vi "Project HMI.vi"() -> ()   [LabVIEW 2025]
panel:
  in  "Statistics":bool
  out "Statistics:":T1
  out "path":path
  out "temp file path":path
  in  "Save":bool
  out "?":T2 {"Temperature °C" scale=0.0..100.0}
  in  "ON/OFF":bool
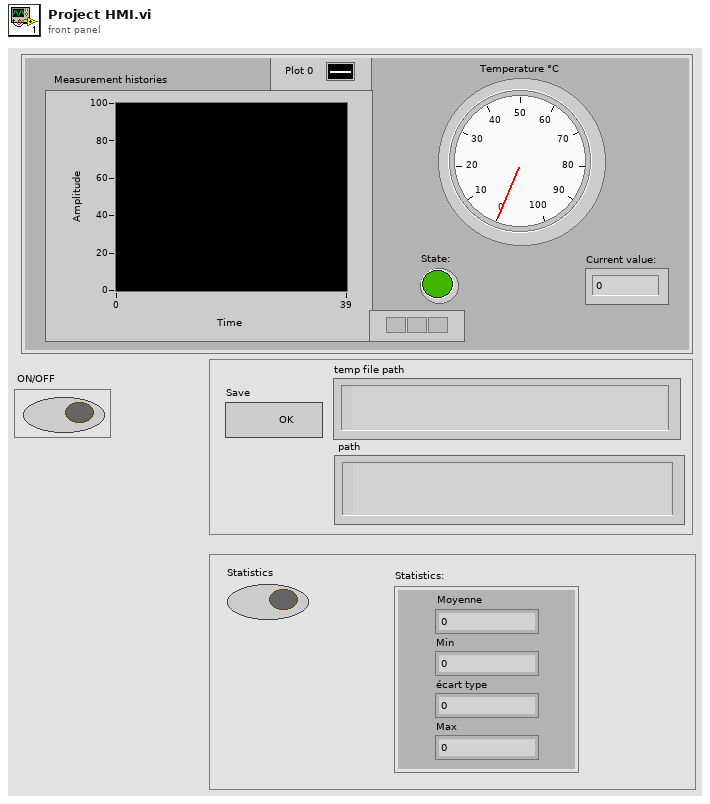
[diagram p1: front panel]
types:
  T1 = cluster{"Moyenne":dbl, "Min":dbl, "écart type":dbl, "Max":dbl}
  T2 = cluster{"Temperature °C":dbl, "Current value:":dbl, "State:":bool, "Measurement histories":dbl}
  T3 = cluster{"Temperature °C":dbl, "Valeur actuelle":dbl, "état:":bool, "Historique des mesures":dbl}
  T4 = enum16{"open", "replace", "create", "open or create", "replace or create", "replace or create with confirmation"}
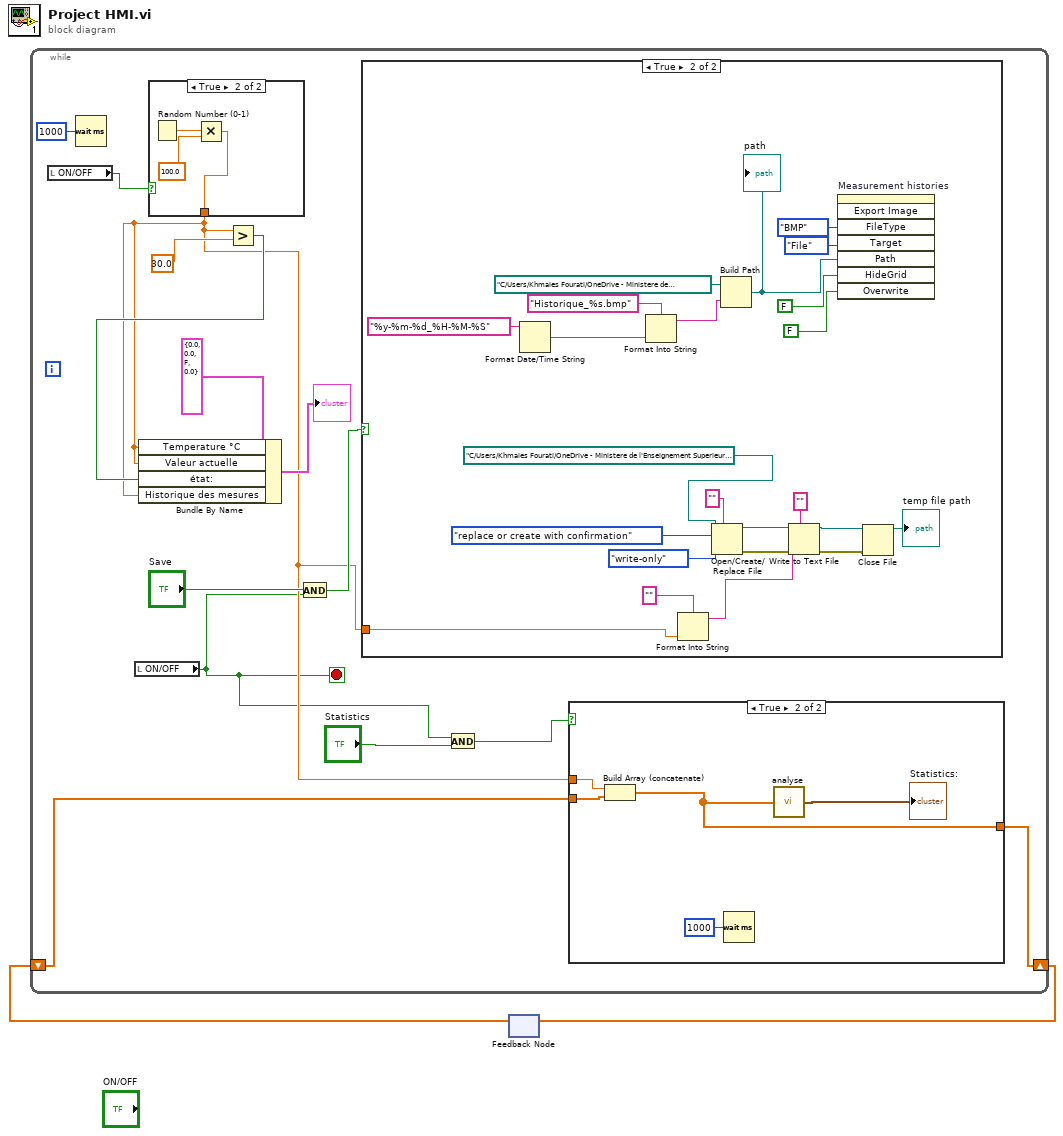
[diagram p0: block diagram]
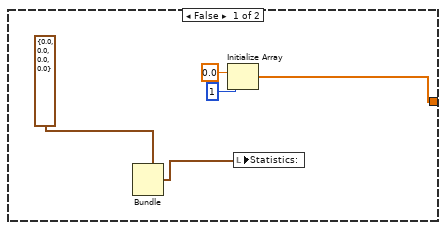
[diagram p2: hidden frame]
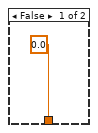
[diagram p4: hidden frame]
diagram:
  n1 = feedback #1() -> (w1:dbl[])  [unwired: 1 in]
  n2 = while {
    shift-right: [w6] -> w2
    shift-left: w1 -> [w7]
    stop <- w5 stop-if-true
    n3 = local read "ON/OFF"() -> (w14:bool)
    n4 = Wait (ms)(milliseconds to wait=u32 1000) -> ()  [unwired: 1 out]
    n5 = local read "ON/OFF"() -> (w5:bool)
    n6 = case shown="True" w14 {
      tunnel: [0.0 w51] -> w8
      frame False {
      }
      frame True {
        n7 = Random Number (0-1)() -> (number: 0 to 1=w53:dbl)
        n8 = Multiply(x=w53, y=100.0) -> (x*y=w51:dbl)
      }
    }
    n9 = Greater?(x=w8, y=30.0) -> (0:w13:bool)
    n10 = Bundle By Name(cluster=T3 {"Temperature °C"=0.0, "Valeur actuelle"=0.0, "état:"=FALSE, "Historique des mesures"=0.0} ("Cluster"), "Temperature °C"=w8, "Valeur actuelle"=w8, "état:"=w13, "Historique des mesures"=w8) -> (→"?":T3)
    n11 = And(x="Save", y=w5) -> (x .and. y?=w9:bool)
    n12 = case shown="True" w9 {
      tunnel: w8 -> [_ w27]
      frame False {
      }
      frame True {
        n13 = Format Date/Time String(time format string (%c)="%y-%m-%d_%H-%M-%S") -> (date/time string=w28:string)  [unwired: 2 in]
        n14 = Format Into String(format string="Historique_%s.bmp", w28) -> (resulting string=w31:string)  [unwired: 2 in, 1 out]
        n15 = Format Into String "Format Into String"(format string="", w27) -> (resulting string=w49:string)  [unwired: 2 in, 1 out]
        n16 = Open/Create/Replace File(file path (use dialog)=path "C:/Users/Khmaies Fourati/OneDrive - Ministere de l'Enseignement Superieur et de la Recherche Scientifique/Documents/LabView projects/mesures.txt", prompt="", operation (0:open)=T4."replace or create with confirmation", access (0:read/write)=enum16{"read/write", "read-only", "write-only"}."write-only") -> (refnum out=w47:refnum<file>, error out=w40:errorcluster)  [unwired: 2 in, 1 out]
        n17 = Build Path(base path=path "C:/Users/Khmaies Fourati/OneDrive - Ministere de l'Enseignement Superieur et de la Recherche Scientifique/Documents/LabView projects", name or relative path=w31) -> (appended path=w34:path)
        "path" <- w34
        n18 = Write to Text File(prompt (Choose or enter file path)="", file (use dialog)=w47, text=w49, error in=w40) -> (refnum out=w42:refnum<file>, error out=w39:errorcluster)  [unwired: 1 out]
        n19 = invoke on="Measurement histories" class="WFChart (strict)" method="Export Image"("FileType"=enum32{"BMP", "EPS", "EMF", "PICT"}."BMP" ("File Type"), "Target"=enum32{"File", "Clipboard"}."File", "Path"=w34, "HideGrid"=FALSE ("Hide Grid"), "Overwrite"=FALSE ("Always Overwrite")) -> ()  [unwired: 3 in, 8 out]
        n20 = Close File(refnum=w42, error in=w39) -> (path=→"temp file path":path)  [unwired: 1 out]
      }
    }
    n21 = And(x=w5, y="Statistics") -> (x .and. y?=w3:bool)
    n22 = case shown="True" w3 {
      tunnel: w8 -> [_ w25]
      tunnel: w7 -> [_ w24]
      tunnel: [w19 w23] -> w6
      frame False {
        n23 = Bundle(cluster=cluster{dbl, dbl, dbl, dbl} {0.0, 0.0, 0.0, 0.0} ("input cluster")) -> (w17:cluster{dbl, dbl, dbl, dbl})  [unwired: 4 in]
        n24 = Initialize Array(0.0 ("element"), 1 ("dimension size")) -> (w19:dbl[])
        n25 = local write "Statistics:"(w17) -> ()
      }
      frame True {
        n26 = Build Array (concatenate)(w25, w24) -> (w23:dbl[])
        n27 = Wait (ms)(milliseconds to wait=u32 1000) -> ()  [unwired: 1 out]
        n28 = call "analyse.vi"("Array"=w23) -> ("Cluster"=→"Statistics:":T1)
      }
    }
  }
  n29 = feedback-in #1(w2) -> ()
